vi "Write Status Reference.vi"(8 "error in (no error)":errorcluster, 10 "Status":T1, 11 "MB_TCP in":refnum<class "MB_TCP.lvclass">) -> (0 "error out":errorcluster, 3 "MB_TCP out":refnum<class "MB_TCP.lvclass">)   [LabVIEW 2019, in "MB_TCP.lvclass"]
uses:
  MB_TCP.lvclass
  Eth Status/Ctl/Status.ctl
  MB_TCP_State.ctl
  MB_TCP.lvclass/MB_TCP.ctl
  Eth Status/Eth Status.lvlib
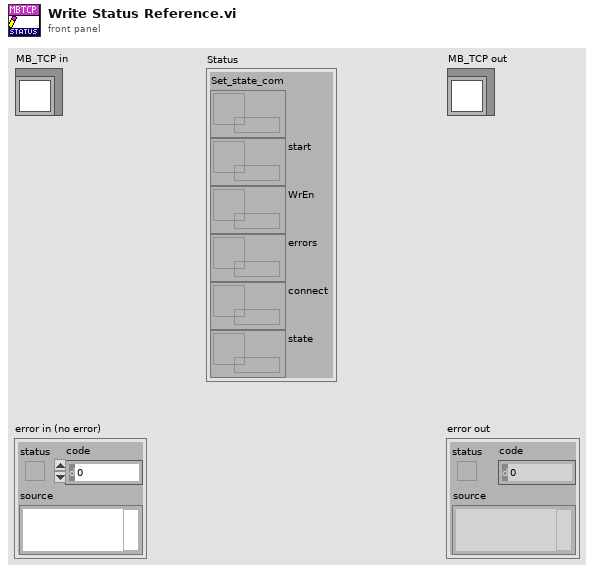
[diagram p1: front panel]
types:
  T1 = typedef "Eth Status.lvlib/Status.ctl" = cluster{"Set_state_com":refnum<data-value>, "start":refnum<data-value>, "WrEn":refnum<data-value>, "errors":refnum<data-value>, "connect":refnum<data-value>, "state":refnum<data-value>}
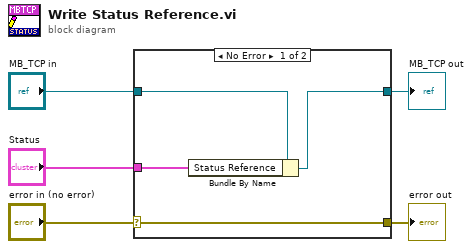
[diagram p0: block diagram]
diagram:
  n1 = case shown="No Error" "error in (no error)" {
    selector: "error in (no error)" -> [w6 w11]
    tunnel: [w6 w11] -> w4
    tunnel: [w8 w10] -> w3
    tunnel: "Status" -> [w7 _]
    tunnel: "MB_TCP in" -> [w9 w10]
    frame No Error {
      n2 = Bundle By Name(cluster=w9, "Status Reference"=w7) -> (w8:refnum<class "MB_TCP.lvclass">)
    }
    frame Error {
    }
  }
  "error out" <- w4
  "MB_TCP out" <- w3
